vi "Add Wheel Speed Sensor card.vi"(8 "error in (no error)":errorcluster, 11 "Node Ptr":u64 format="%.0x") -> (0 "error out":errorcluster)   [LabVIEW 2014, in "SLSC configuration System Explorer.lvlib"]
uses:
  SLSC configuration System Explorer.lvlib
  Shared/Constants.vi
  Shared/SLSC configuration Shared.lvlib
panel:
  in  "Tag":string
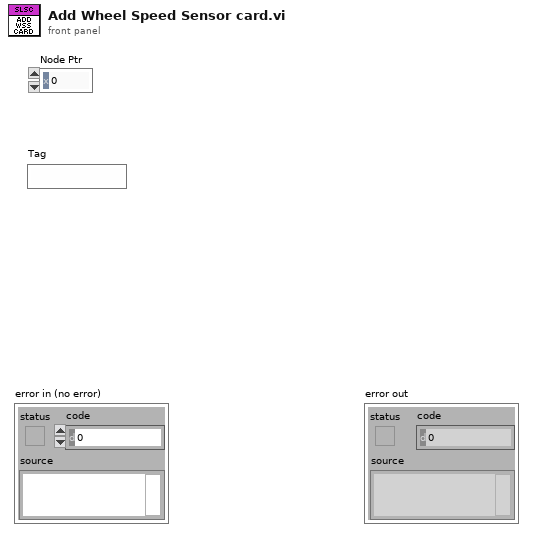
[diagram p1: front panel]
types:
  T1 = typedef "SLSC configuration Shared.lvlib/Card Position.ctl" = cluster{"Rack #":u8, "Slot #":T2}
  T2 = typedef "SLSC configuration Shared.lvlib/Slot #.ctl" = u8
  T3 = typedef "Custom Device API.lvlib/Custom Device Item Ref.ctl" = u64
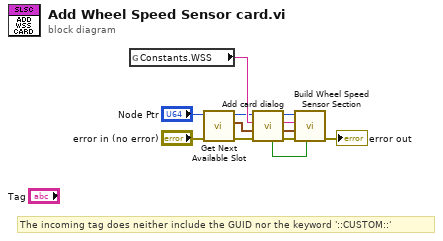
[diagram p0: block diagram]
diagram:
  # "The incoming tag does neither include the GUID nor the keyword '::CUSTOM::'"
  n1 = global read "Constants.vi" "Constants.WSS"() -> (w12:string)
  n2 = call "Get Next Available Slot.vi"("error in (no error)"="error in (no error)", "Device Ref in"="Node Ptr") -> ("error out"=w4:errorcluster, "Next Open Slot"=w1:T1, "Device Ref out"=w2:T3)  [unwired: 7 in]
  n3 = call "Add card dialog.vi"("error in (no error)"=w4, "Card Position"=w1, "Card Type in"=w12, "Node Ptr"=w2) -> ("error out"=w11:errorcluster, "Card Position out"=w9:T1, "Name out"=w7:string, "Node Ptr out"=w10:u64, "Cancelled?"=w6:bool)  [unwired: 3 in]
  n4 = call "Build Wheel Speed Sensor Section.vi"("Cancelled?"=w6, "error in (no error)"=w11, "Card Position in"=w9, "Name in"=w7, "Node Ptr in"=w10) -> ("error out"=→"error out":errorcluster)  [unwired: 6 in]
